vi "Delete Exchanges.vi"(8 "error in (no error)":errorcluster caption="entrée d'erreur (pas d'erreur)", 10 "Position":i32, 11 "Exchanges en entrée":refnum<class "Exchanges.lvclass"> caption="DNL_LabVIEW Object in") -> (0 "error out":errorcluster caption="sortie d'erreur", 3 "Exchanges en sortie":refnum<class "Exchanges.lvclass"> caption="DNL_LabVIEW Object out")   [LabVIEW 2012, in "Exchanges.lvclass"]
uses:
  Exchanges.lvclass
  Exchanges.lvclass/Exchanges.ctl
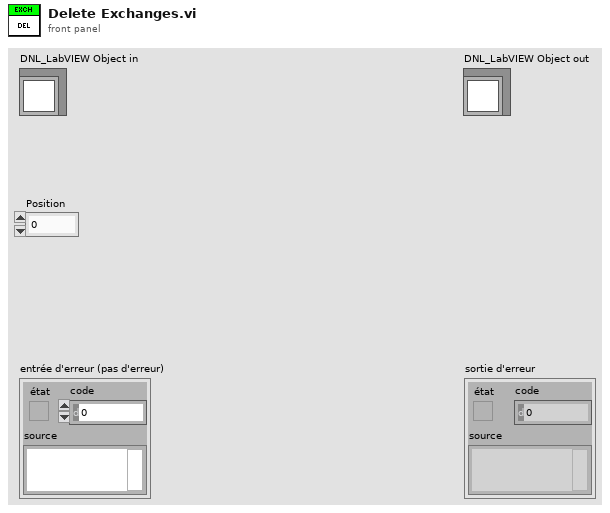
[diagram p1: front panel]
types:
  T1 = typedef "Dictionary Object RefNum__ogtk.ctl" = refnum<k1>
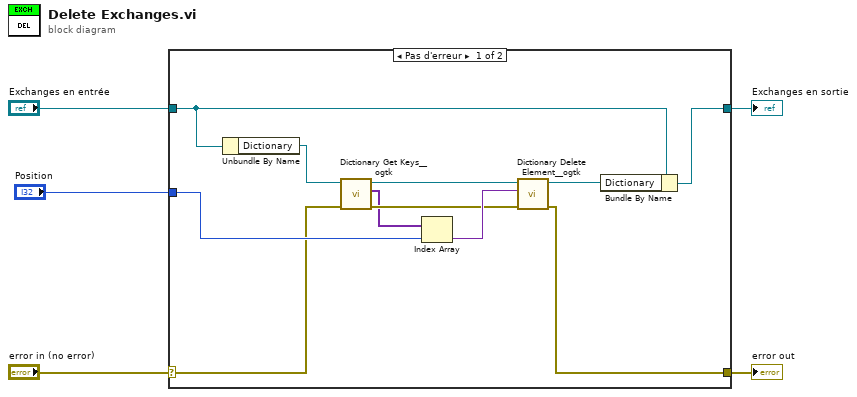
[diagram p0: block diagram]
diagram:
  n1 = case shown="Pas d'erreur" "error in (no error)" {
    selector: "error in (no error)" -> [w6 w18]
    tunnel: [w7 w18] -> w4
    tunnel: [w8 w17] -> w2
    tunnel: "Exchanges en entrée" -> [w9 w17]
    tunnel: "Position" -> [w10 _]
    frame No Error {
      n2 = Unbundle By Name(w9) -> ("Dictionary"=w13:T1)
      n3 = call <userlib>:"Dictionary Get Keys__ogtk.vi"("error in (no error)"=w6, "dictionary"=w13) -> ("error out"=w15:errorcluster, "keys"=w12:variant[], "dictionary out"=w14:T1)  [unwired: 7 in]
      n4 = Index Array(array=w12, index=w10) -> (element=w16:variant)
      n5 = call <userlib>:"Dictionary Delete Element__ogtk.vi"("error in (no error)"=w15, "key"=w16, "dictionary"=w14) -> ("error out"=w7:errorcluster, "dictionary out"=w11:T1)  [unwired: 7 in]
      n6 = Bundle By Name(cluster=w9, "Dictionary"=w11) -> (w8:refnum<class "Exchanges.lvclass">)
    }
    frame Error {
    }
  }
  "error out" <- w4
  "Exchanges en sortie" <- w2
